vi "ThermresistorMarcoGonzalez.vi"() -> ()   [LabVIEW 2012]
panel:
  out "Cold":bool
  out "Warm":bool
  out "Temp (C)":dbl
  out "Temp Chart":dbl(graph)
  in  "stop":bool
  out "Temp (K)":dbl
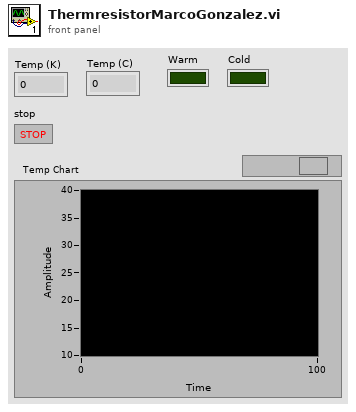
[diagram p1: front panel]
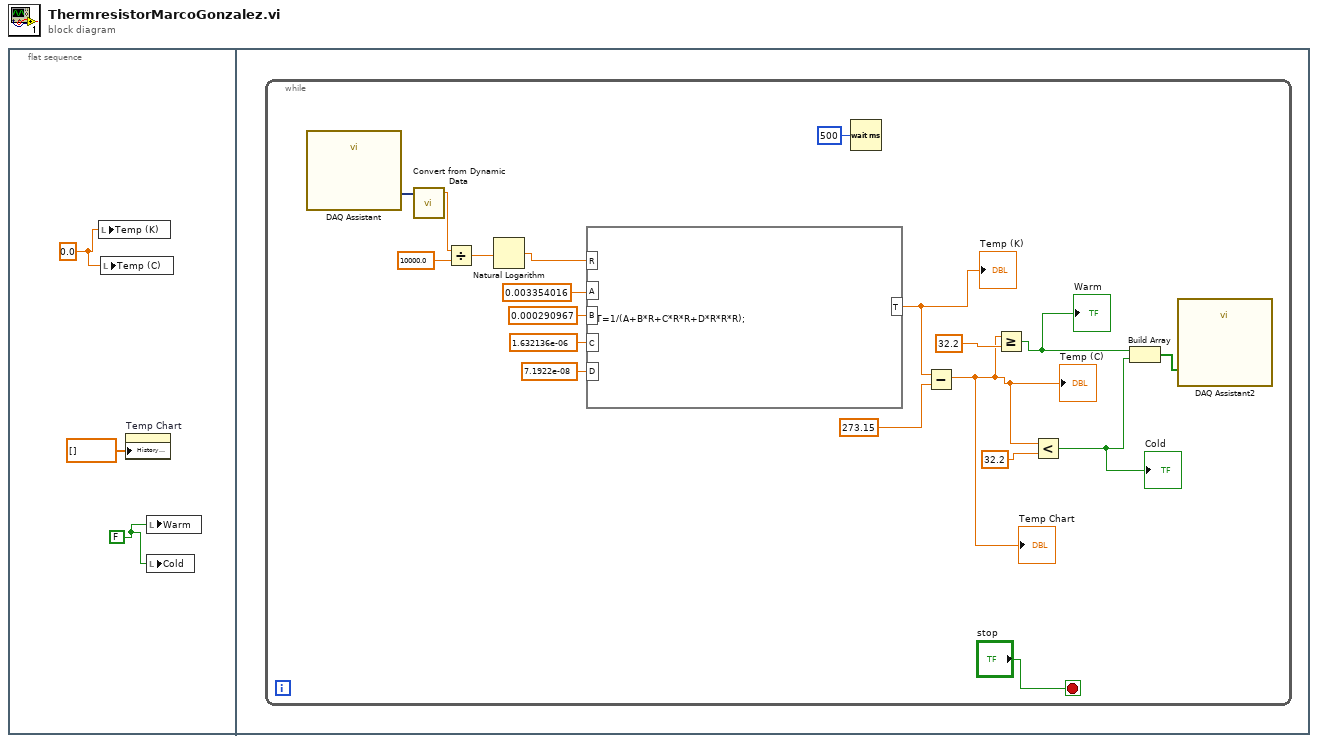
[diagram p0: block diagram]
diagram:
  n1 = flat-sequence {
    frame #0 {
      w1 = FALSE
      w3 = 0.0
      n2 = local write "Temp (K)"(w3) -> ()
      n3 = local write "Temp (C)"(w3) -> ()
      n4 = property on="Temp Chart" class="WFChart (strict)"("History Data"=dbl[] []) -> ()  [unwired: 2 in, 2 out]
      n5 = local write "Warm"(w1) -> ()
      n6 = local write "Cold"(w1) -> ()
    }
    frame #1 {
      n7 = while {
        stop <- "stop" stop-if-true
        n8 = call "DAQ Assistant"() -> ("data"=w13:dynamicdata)  [unwired: 17 in, 2 out]
        n9 = call "Convert from Dynamic Data"("Dynamic Data Type"=w13) -> ("Scalar"=w12:dbl)  [unwired: 3 in]
        n10 = Divide(x=w12, y=10000.0) -> (x/y=w15:dbl)
        n11 = Natural Logarithm(1:w15) -> (0:w11:dbl)
        n12 = formula code="T=1/(A+B*R+C*R*R+D*R*R*R);"("R"=w11, "A"=0.003354016 ("input variable"), "B"=0.000290967 ("input variable"), "C"=1.632136e-06 ("input variable"), "D"=7.1922e-08 ("input variable")) -> ("T"=w10:dbl)
        "Temp (K)" <- w10
        n13 = Wait (ms)(milliseconds to wait=u32 500) -> ()  [unwired: 1 out]
        n14 = Subtract(x=w10, y=273.15) -> (x-y=w8:dbl)
        "Temp Chart" <- w8
        "Temp (C)" <- w8
        n15 = Greater Or Equal?(x=w8, y=32.2) -> (x >= y?=w5:bool)
        "Warm" <- w5
        n16 = Less?(x=w8, y=32.2) -> (x < y?=w4:bool)
        "Cold" <- w4
        n17 = Build Array(w5, w4) -> (w6:bool[])
        n18 = call "DAQ Assistant2"("data"=w6) -> ()  [unwired: 17 in, 2 out]
      }
    }
  }
